vi "Disconnected.vi"(8 "error in (no error)":errorcluster, 10 "InstrumentData":T1, 11 "SinglePhotonInterferenceUI in":refnum<class "SinglePhotonInterferenceUI.lvclass">) -> (0 "error out":errorcluster, 3 "SinglePhotonInterferenceUI out":refnum<class "SinglePhotonInterferenceUI.lvclass">)   [LabVIEW 2023, in "SinglePhotonInterferenceUI.lvlib" / "SinglePhotonInterferenceUI.lvclass"]
uses:
  SinglePhotonInterferenceUI.lvclass
  typedefs/instrumentType.ctl
  typedefs/typedefs.lvlib
  typedefs/InstrumentData.ctl
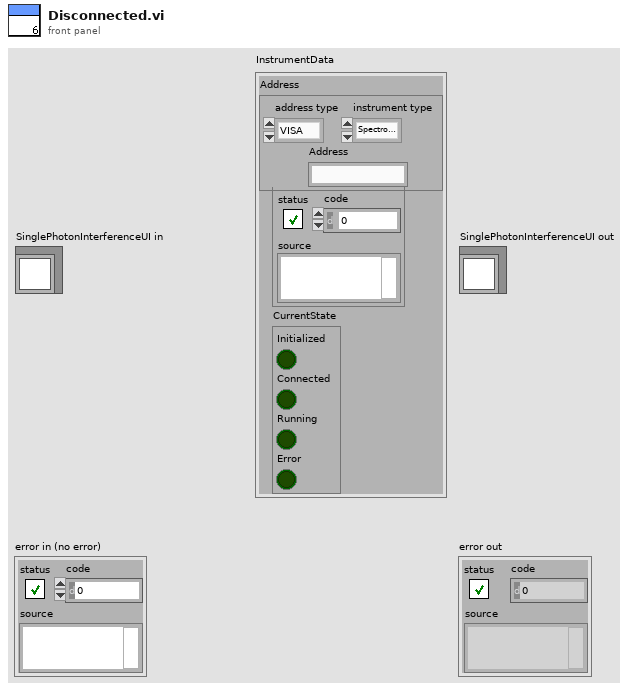
[diagram p1: front panel]
types:
  T1 = typedef "typedefs.lvlib/InstrumentData.ctl" = cluster{"Instr Error":errorcluster, "Address":cluster{"address type":enum16{"VISA", "Index"}, "Address":string, "instrument type":T2}, "CurrentState":cluster{"Initialized":bool, "Connected":bool, "Running":bool, "Error":bool}}
  T2 = typedef "typedefs.lvlib/instrumentType.ctl" = enum16{"Spectrometer", "Camera", "Stepper", "Piezo", "SLM"}
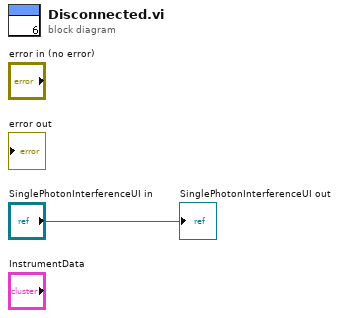
[diagram p0: block diagram]
diagram:
  "SinglePhotonInterferenceUI out" <- "SinglePhotonInterferenceUI in"
